vi "Tell Parent Inspect.vi"(4 "Msg":refnum<class "Msg.lvclass">, 6 "Within Unified Msgs":bool, 8 "Error in":errorcluster, 11 "TEMPLATE Actor in":refnum<class "TEMPLATE Actor.lvclass">) -> (0 "Error out":errorcluster, 2 "Proceed":bool=TRUE, 3 "TEMPLATE Actor out":refnum<class "TEMPLATE Actor.lvclass">)   [LabVIEW 2020, in "_Template.lvlib" / "Templates.lvlib" / "TEMPLATE jettl Actor.lvlib" / "TEMPLATE Actor.lvlib" / "TEMPLATE Actor.lvclass"]
uses:
  TEMPLATE Actor.lvclass
  C:/git/jettl/src/jettl/jettl/Actor/Actor.lvclass
  jettl/jettl/Msg/Msg.lvclass
  jettl/jettl/Actor/Actor.lvclass
  TEMPLATE Actor.lvclass/TEMPLATE Actor.ctl
  jettl/jettl/jettl.lvlib
panel:
  # "This front panel should not be manipulated."
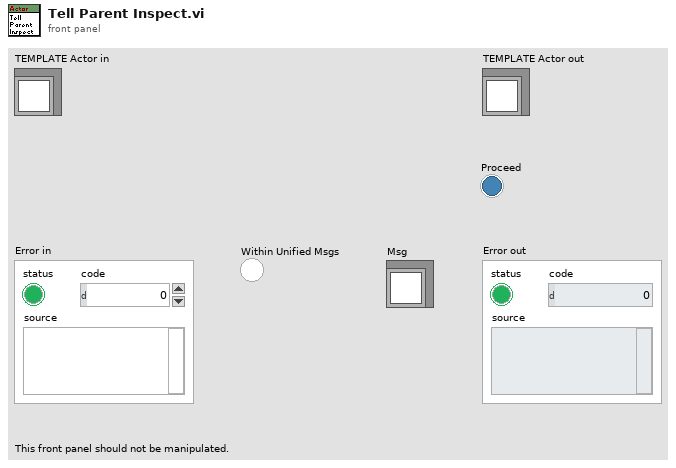
[diagram p1: front panel]
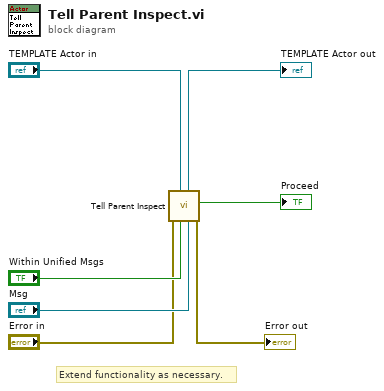
[diagram p0: block diagram]
diagram:
  # "Extend functionality as necessary."
  n1 = call "Tell Parent Inspect.vi"("Msg"="Msg", "Within Unified Msgs"="Within Unified Msgs", "Actor in"="TEMPLATE Actor in", "Error in"="Error in") -> ("Error out"=→"Error out":errorcluster, "Proceed"=→"Proceed":bool, "Actor out"=→"TEMPLATE Actor out":refnum<class "TEMPLATE Actor.lvclass">)  [unwired: 5 in]
